vi "Add Channel Properties To String Array.vi"(8 "error in":errorcluster, 10 "Properties List In":string[][](array[string]), 11 "Channel Ref in":T1 format="%.0x") -> (0 "error out":errorcluster, 2 "Properties List Out":string[][](array[string]), 3 "Channel Ref out":T1 format="%.0x")   [LabVIEW 2017, in "PXImc System Explorer.lvlib"]
uses:
  PXImc System Explorer.lvlib
  <vilib>/NI Veristand/Custom Device API/Custom Device Item Ref.ctl
  NationalInstruments.VeriStand.SystemDefinitionAPI
  NationalInstruments.VeriStand.SystemStorage
  <vilib>/NI VeriStand/Custom Device API/Custom Device API.lvlib
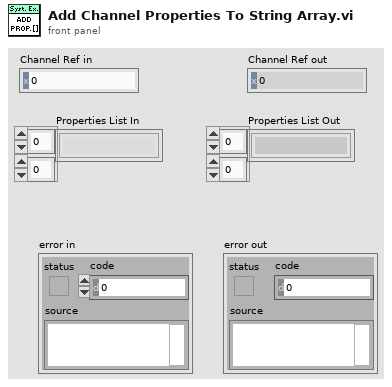
[diagram p1: front panel]
types:
  T1 = typedef "Custom Device API.lvlib/Custom Device Item Ref.ctl" = u64
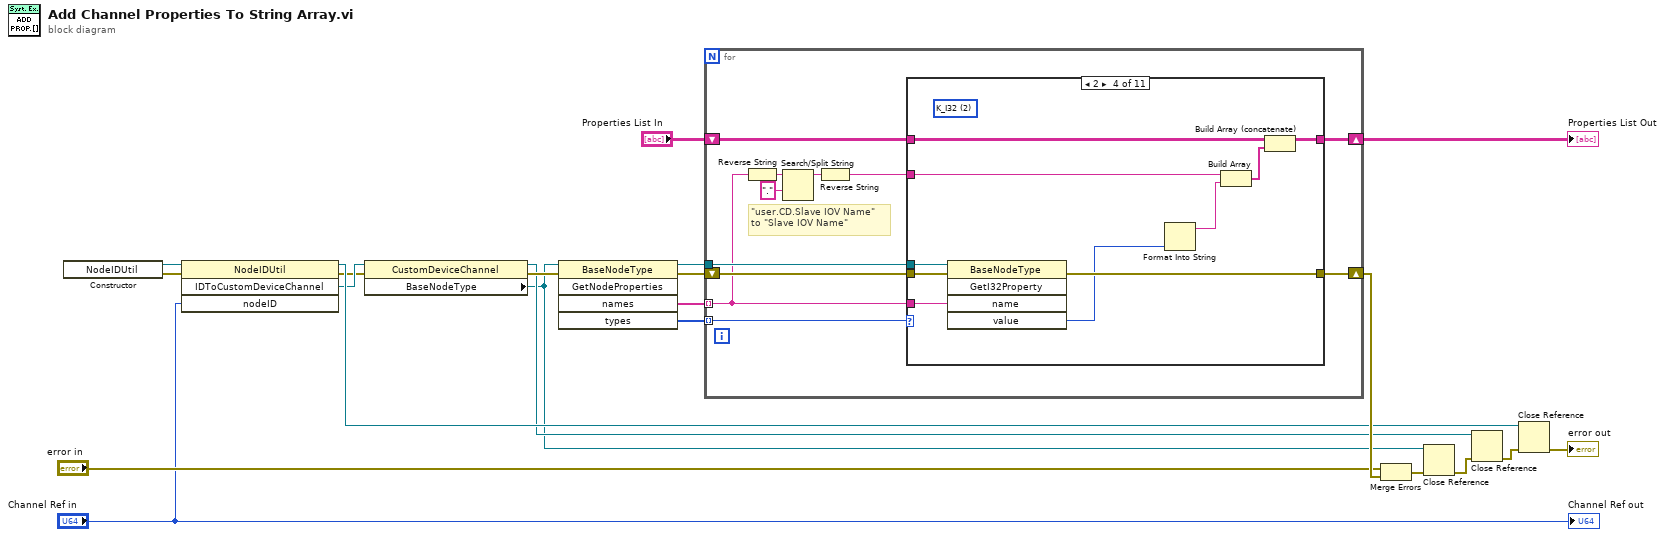
[diagram p0: block diagram]
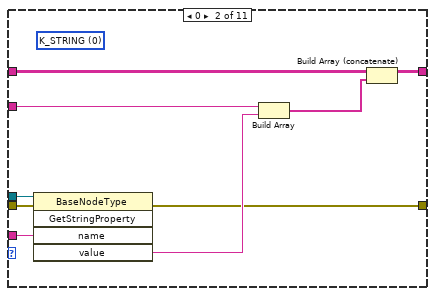
[diagram p3: hidden frame]
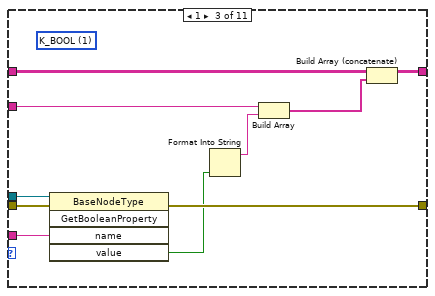
[diagram p4: hidden frame]
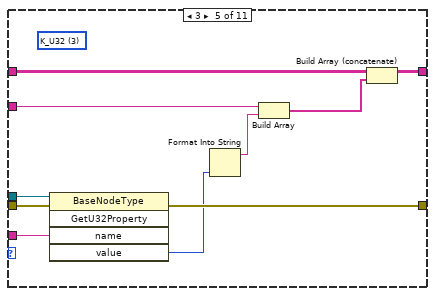
[diagram p5: hidden frame]
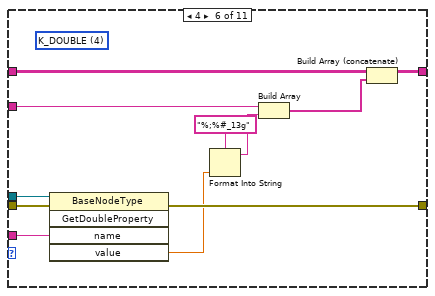
[diagram p6: hidden frame]
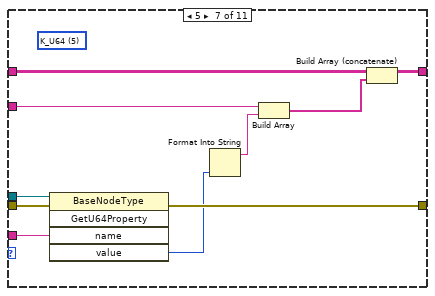
[diagram p7: hidden frame]
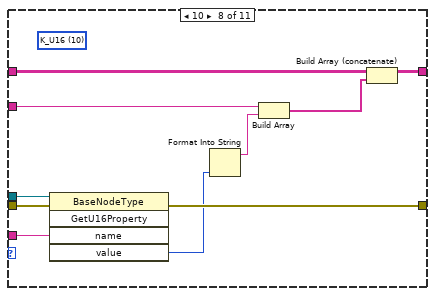
[diagram p8: hidden frame]
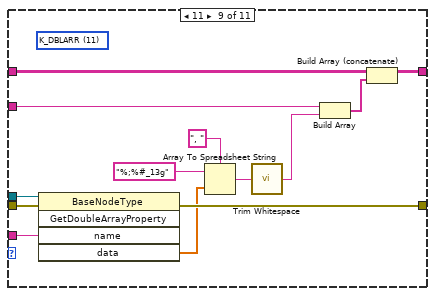
[diagram p9: hidden frame]
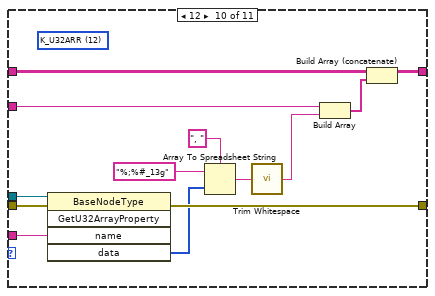
[diagram p10: hidden frame]
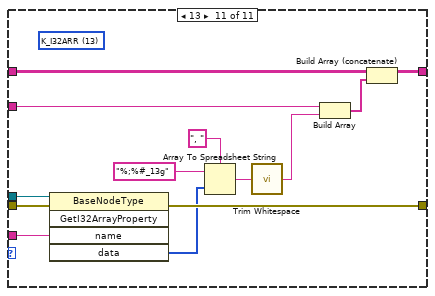
[diagram p11: hidden frame]
diagram:
  n1 = constructor class="NodeIDUtil"() -> (reference out=w14:refnum<k24>, error out=w13:errorcluster)  [unwired: 3 in, 1 out]
  n2 = invoke class="NodeIDUtil" method="IDToCustomDeviceChannel"(reference=w14, error in=w13, "nodeID"="Channel Ref in") -> (reference out=w12:refnum<k24>, error out=w10:errorcluster, "IDToCustomDeviceChannel"=w11:refnum<k24>)  [unwired: 1 in, 1 out]
  n3 = property class="CustomDeviceChannel"(reference=w11, error in=w10) -> (reference out=w8:refnum<k24>, error out=w9:errorcluster, "BaseNodeType"=w3:refnum<k24>)
  n4 = invoke class="BaseNodeType" method="GetNodeProperties"(reference=w3, error in=w9) -> (reference out=w20:refnum<k24>, error out=w15:errorcluster, "names"=w19:string[], "types"=w21:i32[])  [unwired: 3 in, 1 out]
  n5 = for {
    shift-right: [w30] -> w18
    shift-left: w15 -> [w28]
    tunnel: w19 -> [w23] mode=indexing
    shift-right: [w32] -> w17
    shift-left: "Properties List In" -> [w31]
    tunnel: w21 -> [w22] mode=indexing
    tunnel: w20 -> [w29]
    # "\"user.CD.Slave IOV Name\"\nto \"Slave IOV Name\""
    n6 = Reverse String(1:w23) -> (0:w27:string)
    n7 = Search/Split String(string=w27, search string/char (-)=".") -> (substring before match=w26:string)  [unwired: 1 in, 2 out]
    n8 = Reverse String(1:w26) -> (0:w24:string)
    n9 = case shown="2" w22 {
      tunnel: [w34 w37 w48 w59 w68 w79 w89 w99 w112 w125 w138] -> w32
      tunnel: w31 -> [w34 w43 w53 w63 w73 w84 w94 w104 w117 w130 w143]
      tunnel: [w33 w38 w49 w60 w69 w80 w90 w100 w113 w126 w139] -> w30
      tunnel: w23 -> [_ w40 w50 w56 w70 w81 w91 w101 w114 w127 w140]
      tunnel: w29 -> [_ w42 w52 w62 w72 w83 w93 w103 w116 w129 w142]
      tunnel: w28 -> [w33 w41 w51 w61 w71 w82 w92 w102 w115 w128 w141]
      tunnel: w24 -> [_ w35 w44 w55 w64 w74 w85 w95 w105 w118 w131]
      frame Default {
      }
      frame 0 {
        (unwired) 0 items=["K_STRING", "K_BOOL", "K_I32", "K_U32", "K_DOUBLE", "K_U64", "K_VARIANT", "K_DEPENDENTFILE", "K_DEPENDENTNODE", "K_DATASOURCENODE", "K_U16", "K_DBLARR", "K_U32ARR", "K_I32ARR"]
        n10 = invoke class="BaseNodeType" method="GetStringProperty"(reference=w42, error in=w41, "name"=w40) -> (error out=w38:errorcluster, "value"=w39:string)  [unwired: 2 in, 3 out]
        n11 = Build Array(w35, w39) -> (w36:string[])
        n12 = Build Array (concatenate)(w43, w36) -> (w37:string[][])
      }
      frame 1 {
        (unwired) 1 items=["K_STRING", "K_BOOL", "K_I32", "K_U32", "K_DOUBLE", "K_U64", "K_VARIANT", "K_DEPENDENTFILE", "K_DEPENDENTNODE", "K_DATASOURCENODE", "K_U16", "K_DBLARR", "K_U32ARR", "K_I32ARR"]
        n13 = invoke class="BaseNodeType" method="GetBooleanProperty"(reference=w52, error in=w51, "name"=w50) -> (error out=w49:errorcluster, "value"=w46:bool)  [unwired: 2 in, 3 out]
        n14 = Format Into String(w46) -> (resulting string=w45:string)  [unwired: 3 in, 1 out]
        n15 = Build Array(w44, w45) -> (w47:string[])
        n16 = Build Array (concatenate)(w53, w47) -> (w48:string[][])
      }
      frame 2 {
        (unwired) 2 items=["K_STRING", "K_BOOL", "K_I32", "K_U32", "K_DOUBLE", "K_U64", "K_VARIANT", "K_DEPENDENTFILE", "K_DEPENDENTNODE", "K_DATASOURCENODE", "K_U16", "K_DBLARR", "K_U32ARR", "K_I32ARR"]
        n17 = invoke class="BaseNodeType" method="GetI32Property"(reference=w62, error in=w61, "name"=w56) -> (error out=w60:errorcluster, "value"=w57:i32)  [unwired: 2 in, 3 out]
        n18 = Format Into String(w57) -> (resulting string=w54:string)  [unwired: 3 in, 1 out]
        n19 = Build Array(w55, w54) -> (w58:string[])
        n20 = Build Array (concatenate)(w63, w58) -> (w59:string[][])
      }
      frame 3 {
        (unwired) 3 items=["K_STRING", "K_BOOL", "K_I32", "K_U32", "K_DOUBLE", "K_U64", "K_VARIANT", "K_DEPENDENTFILE", "K_DEPENDENTNODE", "K_DATASOURCENODE", "K_U16", "K_DBLARR", "K_U32ARR", "K_I32ARR"]
        n21 = invoke class="BaseNodeType" method="GetU32Property"(reference=w72, error in=w71, "name"=w70) -> (error out=w69:errorcluster, "value"=w66:u32)  [unwired: 2 in, 3 out]
        n22 = Format Into String(w66) -> (resulting string=w65:string)  [unwired: 3 in, 1 out]
        n23 = Build Array(w64, w65) -> (w67:string[])
        n24 = Build Array (concatenate)(w73, w67) -> (w68:string[][])
      }
      frame 4 {
        (unwired) 4 items=["K_STRING", "K_BOOL", "K_I32", "K_U32", "K_DOUBLE", "K_U64", "K_VARIANT", "K_DEPENDENTFILE", "K_DEPENDENTNODE", "K_DATASOURCENODE", "K_U16", "K_DBLARR", "K_U32ARR", "K_I32ARR"]
        n25 = invoke class="BaseNodeType" method="GetDoubleProperty"(reference=w83, error in=w82, "name"=w81) -> (error out=w80:errorcluster, "value"=w77:dbl)  [unwired: 2 in, 3 out]
        n26 = Format Into String(format string="%;%#_13g", w77) -> (resulting string=w76:string)  [unwired: 2 in, 1 out]
        n27 = Build Array(w74, w76) -> (w78:string[])
        n28 = Build Array (concatenate)(w84, w78) -> (w79:string[][])
      }
      frame 5 {
        (unwired) 5 items=["K_STRING", "K_BOOL", "K_I32", "K_U32", "K_DOUBLE", "K_U64", "K_VARIANT", "K_DEPENDENTFILE", "K_DEPENDENTNODE", "K_DATASOURCENODE", "K_U16", "K_DBLARR", "K_U32ARR", "K_I32ARR"]
        n29 = invoke class="BaseNodeType" method="GetU64Property"(reference=w93, error in=w92, "name"=w91) -> (error out=w90:errorcluster, "value"=w87:u64)  [unwired: 2 in, 3 out]
        n30 = Format Into String(w87) -> (resulting string=w86:string)  [unwired: 3 in, 1 out]
        n31 = Build Array(w85, w86) -> (w88:string[])
        n32 = Build Array (concatenate)(w94, w88) -> (w89:string[][])
      }
      frame 10 {
        (unwired) 10 items=["K_STRING", "K_BOOL", "K_I32", "K_U32", "K_DOUBLE", "K_U64", "K_VARIANT", "K_DEPENDENTFILE", "K_DEPENDENTNODE", "K_DATASOURCENODE", "K_U16", "K_DBLARR", "K_U32ARR", "K_I32ARR"]
        n33 = invoke class="BaseNodeType" method="GetU16Property"(reference=w103, error in=w102, "name"=w101) -> (error out=w100:errorcluster, "value"=w97:u16)  [unwired: 2 in, 3 out]
        n34 = Format Into String(w97) -> (resulting string=w96:string)  [unwired: 3 in, 1 out]
        n35 = Build Array(w95, w96) -> (w98:string[])
        n36 = Build Array (concatenate)(w104, w98) -> (w99:string[][])
      }
      frame 11 {
        (unwired) 11 items=["K_STRING", "K_BOOL", "K_I32", "K_U32", "K_DOUBLE", "K_U64", "K_VARIANT", "K_DEPENDENTFILE", "K_DEPENDENTNODE", "K_DATASOURCENODE", "K_U16", "K_DBLARR", "K_U32ARR", "K_I32ARR"]
        n37 = invoke class="BaseNodeType" method="GetDoubleArrayProperty"(reference=w116, error in=w115, "name"=w114) -> (error out=w113:errorcluster, "data"=w110:dbl[])  [unwired: 2 in, 3 out]
        n38 = Array To Spreadsheet String(delimiter (Tab)=", ", array=w110, 3:"%;%#_13g" ("format string")) -> (spreadsheet string=w109:string)
        n39 = call <vilib>:"Trim Whitespace.vi"("string"=w109) -> ("trimmed string"=w108:string)  [unwired: 1 in]
        n40 = Build Array(w105, w108) -> (w111:string[])
        n41 = Build Array (concatenate)(w117, w111) -> (w112:string[][])
      }
      frame 12 {
        (unwired) 12 items=["K_STRING", "K_BOOL", "K_I32", "K_U32", "K_DOUBLE", "K_U64", "K_VARIANT", "K_DEPENDENTFILE", "K_DEPENDENTNODE", "K_DATASOURCENODE", "K_U16", "K_DBLARR", "K_U32ARR", "K_I32ARR"]
        n42 = invoke class="BaseNodeType" method="GetU32ArrayProperty"(reference=w129, error in=w128, "name"=w127) -> (error out=w126:errorcluster, "data"=w123:u32[])  [unwired: 2 in, 3 out]
        n43 = Array To Spreadsheet String(delimiter (Tab)=", ", array=w123, 3:"%;%#_13g" ("format string")) -> (spreadsheet string=w122:string)
        n44 = call <vilib>:"Trim Whitespace.vi"("string"=w122) -> ("trimmed string"=w121:string)  [unwired: 1 in]
        n45 = Build Array(w118, w121) -> (w124:string[])
        n46 = Build Array (concatenate)(w130, w124) -> (w125:string[][])
      }
      frame 13 {
        (unwired) 13 items=["K_STRING", "K_BOOL", "K_I32", "K_U32", "K_DOUBLE", "K_U64", "K_VARIANT", "K_DEPENDENTFILE", "K_DEPENDENTNODE", "K_DATASOURCENODE", "K_U16", "K_DBLARR", "K_U32ARR", "K_I32ARR"]
        n47 = invoke class="BaseNodeType" method="GetI32ArrayProperty"(reference=w142, error in=w141, "name"=w140) -> (error out=w139:errorcluster, "data"=w136:i32[])  [unwired: 2 in, 3 out]
        n48 = Array To Spreadsheet String(delimiter (Tab)=", ", array=w136, 3:"%;%#_13g" ("format string")) -> (spreadsheet string=w135:string)
        n49 = call <vilib>:"Trim Whitespace.vi"("string"=w135) -> ("trimmed string"=w134:string)  [unwired: 1 in]
        n50 = Build Array(w131, w134) -> (w137:string[])
        n51 = Build Array (concatenate)(w143, w137) -> (w138:string[][])
      }
    }
  }
  "Properties List Out" <- w17
  n52 = Merge Errors("error in", w18) -> (w2:errorcluster)
  n53 = Close Reference(reference=w3, error in (no error)=w2) -> (error out=w4:errorcluster)
  n54 = Close Reference(reference=w8, error in (no error)=w4) -> (error out=w7:errorcluster)
  n55 = Close Reference(reference=w12, error in (no error)=w7) -> (error out=→"error out":errorcluster)
  "Channel Ref out" <- "Channel Ref in"
